vi "Get Slot Bus Device Function.vi"(7 "dwFunction":u32, 9 "dwDevice":u32, 10 "dwBus":u32, 11 "dwslot":u32) -> (1 "dwDevice out":u32, 2 "dwBus out":u32, 3 "dwslot out":u32, 4 "function return":u32, 5 "dwFunction out":u32)   [LabVIEW 2018, in "Copy of Andor SDK.lvlib"]
doc: "EXPNETTYPE unsigned int WINAPI GetSlotBusDeviceFunction(DWORD * dwslot, DWORD * dwBus, DWORD * dwDevice, DWORD * dwFunction);"
uses:
  Copy of Andor SDK.lvlib
  <userlib>/Andor SDK/ATMCD32D.dll
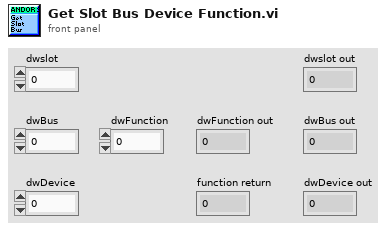
[diagram p1: front panel]
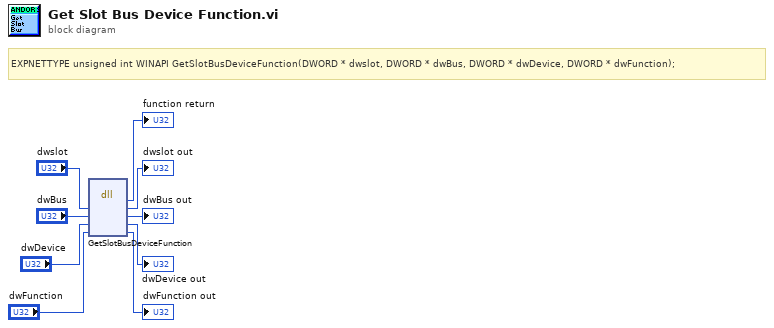
[diagram p0: block diagram]
diagram:
  # "EXPNETTYPE unsigned int WINAPI GetSlotBusDeviceFunction(DWORD * dwslot, DWORD * dwBus, DWORD * dwDevice, DWORD * dwFunction);"
  n1 = dll-call lib="C:/Program Files (x86)/National Instruments/LabVIEW 2018/user.lib/Andor SDK/ATMCD32D.*" fn="GetSlotBusDeviceFunction"("dwslot"="dwslot", "dwBus"="dwBus", "dwDevice"="dwDevice", "dwFunction"="dwFunction") -> (→"function return":u32, "dwslot"=→"dwslot out":u32, "dwBus"=→"dwBus out":u32, "dwDevice"=→"dwDevice out":u32, "dwFunction"=→"dwFunction out":u32)  [unwired: 3 in, 2 out]
